vi "Single_Wire_Magnetic_Field.vi"() -> ()   [LabVIEW 2018]
panel:
  in  "Current":dbl
  in  "Length":dbl
  out "output variable":dbl[][](array[numeric])
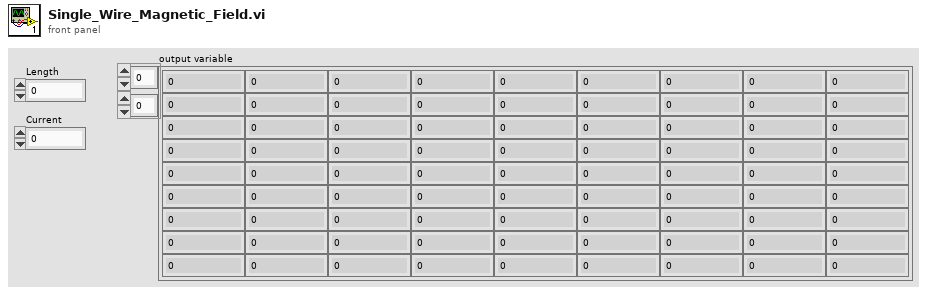
[diagram p1: front panel]
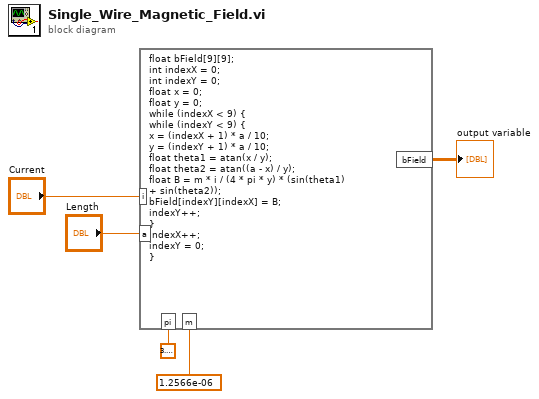
[diagram p0: block diagram]
diagram:
  n1 = formula code="float bField[9][9];\nint indexX = 0;\nint indexY = 0;\nfloat x = 0;\nfloat y = 0;\nwhile (indexX < 9) {\nwhile (indexY < 9) {\nx = (indexX + 1) * a / 10;\ny = (indexY + 1) * a / 10;\nfloat theta1 = atan(x / y);\nfloat theta2 = atan((a - x) / y);\nfloat B = m * i / (4 * pi * y) * (sin(theta1)\n+ sin(theta2));\nbField[indexY][indexX] = B;\nindexY++;\n}\nindexX++;\nindexY = 0;\n}"("i"="Current", "a"="Length", "pi"=3.141592653589793, "m"=1.2566e-06) -> ("bField"=→"output variable":dbl[][])
